vi "setToHex.vi"(1 "Pset":sgl, 2 "Iset":sgl, 3 "Uset":sgl) -> (0 "string":string)   [LabVIEW 2015]
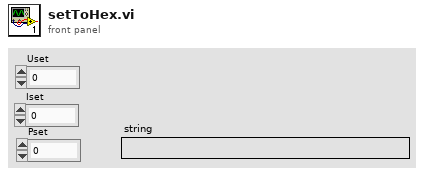
[diagram p1: front panel]
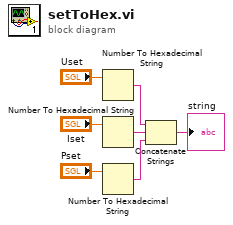
[diagram p0: block diagram]
diagram:
  n1 = Number To Hexadecimal String(2:"Uset") -> (0:w6:string)  [unwired: 1 in]
  n2 = Number To Hexadecimal String(2:"Iset") -> (0:w3:string)  [unwired: 1 in]
  n3 = Number To Hexadecimal String(2:"Pset") -> (0:w2:string)  [unwired: 1 in]
  n4 = Concatenate Strings(w6, w3, w2) -> (→"string":string)
